vi "Filter Mixed Mode Data.vi"(10 "Data":dbl[][](array[numeric])) -> (2 "Mixed Mode Data":T1[](array[typedef]))   [LabVIEW 2009]
uses:
  MixedMode/Mixed Mode Cartesian Data.ctl
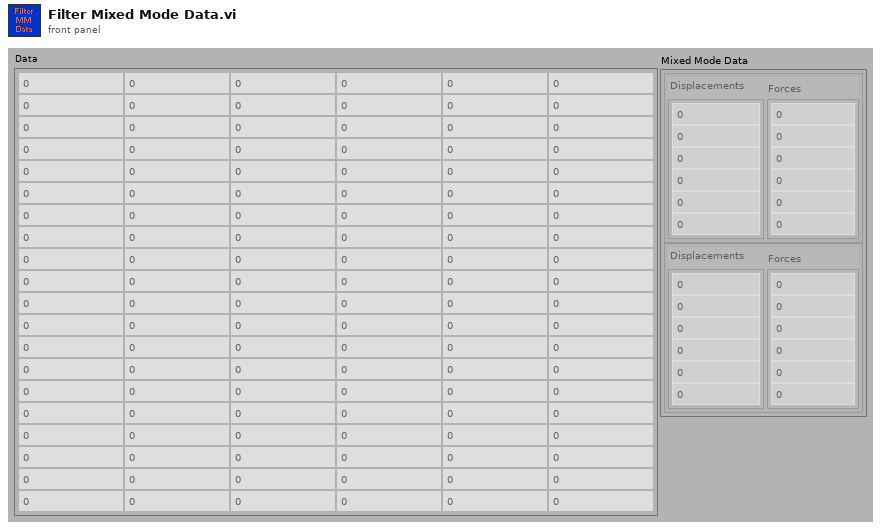
[diagram p1: front panel]
types:
  T1 = typedef "Mixed Mode Cartesian Data.ctl" = cluster{"Displacements":dbl[], "Forces":dbl[]}
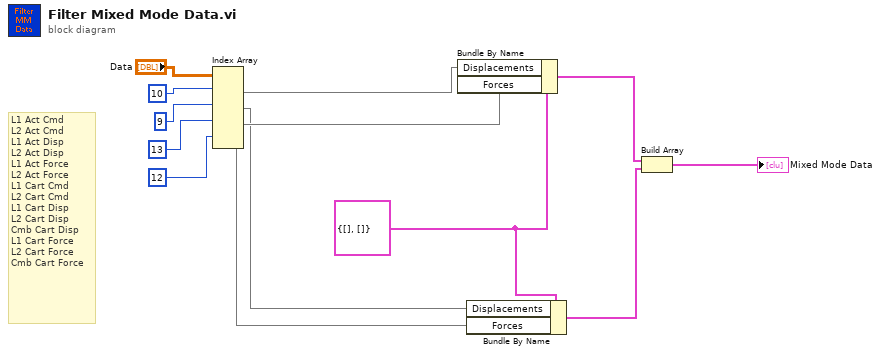
[diagram p0: block diagram]
diagram:
  w13 = T1 {"Displacements"=[], "Forces"=[]} ("LBCB 1 Measurements")
  # "L1 Act Cmd\nL2 Act Cmd\nL1 Act Disp\nL2 Act Disp\nL1 Act Force\nL2 Act Force\nL1 Cart Cmd\nL2 Cart Cmd\nL1 Cart Disp\nL2 Cart Disp\nCmb Cart Disp\nL1 Cart Force\nL2 Cart Force\nCmb Cart Force"
  n1 = Index Array(array="Data", index (row) #1=10 ("index (row)"), index (row) #2=9 ("index (row)"), index (row) #3=13 ("index (row)"), index (row) #4=12 ("index (row)")) -> (element #1=w7:dbl[], element #2=w5:dbl[], element #3=w6:dbl[], element #4=w4:dbl[])  [unwired: 4 in]
  n2 = Bundle By Name(cluster=w13, "Displacements"=w7, "Forces"=w6) -> (w3:T1)
  n3 = Bundle By Name(cluster=w13, "Displacements"=w5, "Forces"=w4) -> (w2:T1)
  n4 = Build Array(w3, w2) -> (→"Mixed Mode Data":T1[])
